vi "Send Batch Messages To Specific Target.vi"(6 "Paras In":variant, 7 "Priority":i32, 8 "error in (no error)":errorcluster, 9 "Mail Strategy In":refnum<class "Mail Strategy.lvclass">, 10 "Messages In":refnum<class "Message.lvclass">[](array[class]), 11 "Map Tree Queue Messenger in":refnum<class "Map Tree Queue Messenger.lvclass">) -> (0 "error out":errorcluster, 3 "Map Tree Queue Messenger out":refnum<class "Map Tree Queue Messenger.lvclass">)   [LabVIEW 2024, in "Map Tree Queue Messenger.lvclass"]
uses:
  Map Tree Queue Messenger.lvclass
  Ancestor Class/Message/Message.lvclass
  Ancestor Class/Messenger/Mail Strategy/Mail Strategy.lvclass
  Mailman/Simple Tree Queue Mailman/Simple Tree Queue Mailman.lvclass
  Ancestor Class/Messenger/Messenger Map Composite/Messenger Map Composite.lvclass/Messenger Map Composite.ctl
  Mailman/Simple Tree Queue Mailman/Simple Tree Queue Mailman.lvclass/Simple Tree Queue Mailman.ctl
  Map Tree Queue Messenger.lvclass/Map Tree Queue Messenger.ctl
  Mailman/Simple Tree Queue Mailman/Public Data/Write Address Recursive Access.vi
  Ancestor Class/Messenger/Messenger Map Composite/Public Data/Read Child Nodes.vi
  Ancestor Class/Messenger/Messenger/Messenger.lvclass
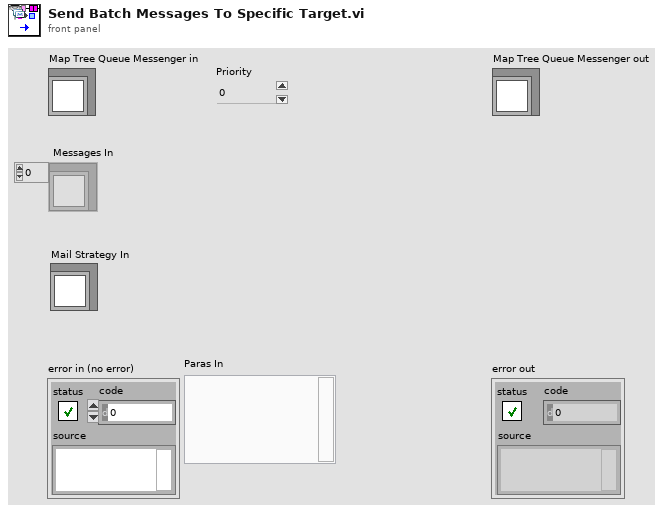
[diagram p1: front panel]
types:
  T1 = typedef "Message Queue.ctl" = refnum<queue>
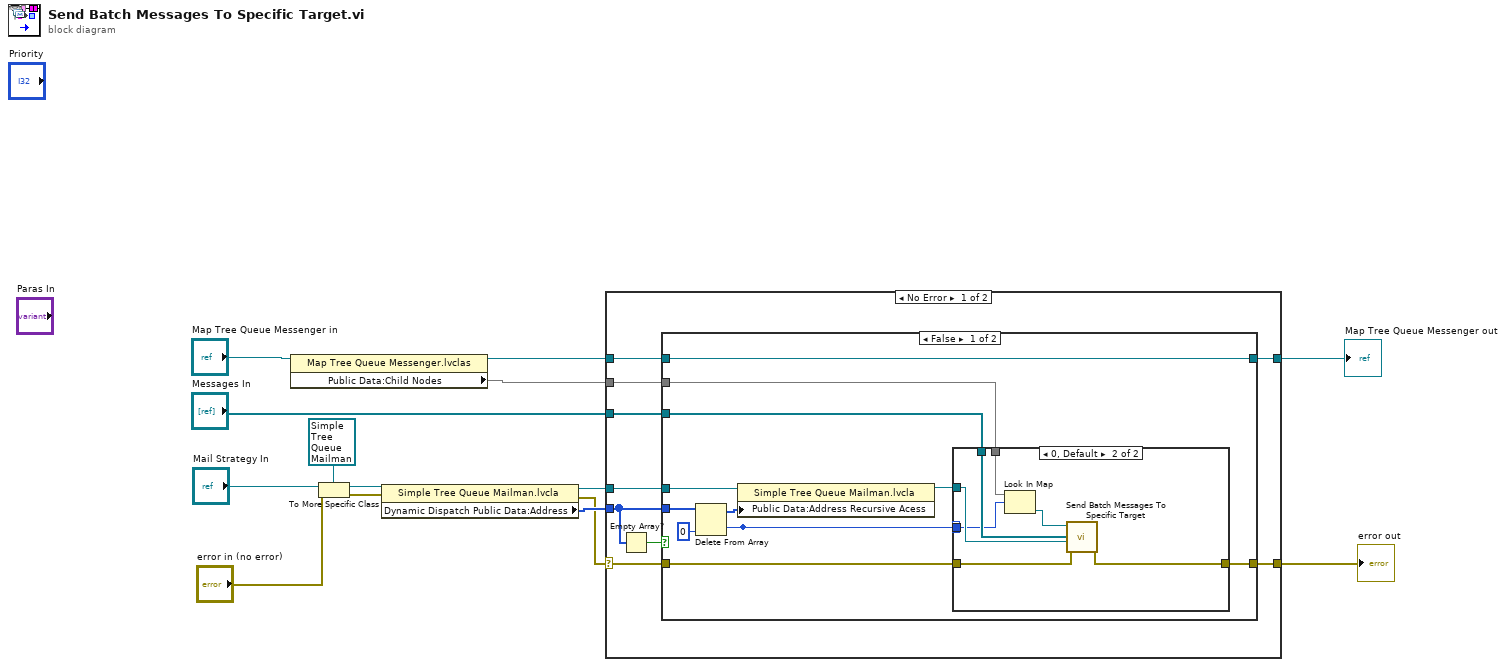
[diagram p0: block diagram]
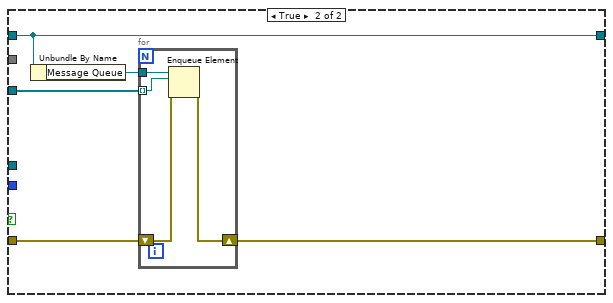
[diagram p3: hidden frame]
diagram:
  n1 = property class="Map Tree Queue Messenger.lvclas"(reference="Map Tree Queue Messenger in") -> (reference out=w9:refnum<class "Map Tree Queue Messenger.lvclass">, "Public Data:Child Nodes"=w8:map{i64, refnum<class "Messenger.lvclass">})  [unwired: 1 in, 1 out]
  n2 = To More Specific Class(target class=refnum<class "Simple Tree Queue Mailman.lvclass"> refnum ("Array Location Mailman.lvclass"), reference="Mail Strategy In", error in="error in (no error)") -> (specific class reference=w12:refnum<class "Simple Tree Queue Mailman.lvclass">, error out=w13:errorcluster)
  n3 = property class="Simple Tree Queue Mailman.lvcla"(reference=w12, error in=w13) -> (reference out=w7:refnum<class "Simple Tree Queue Mailman.lvclass">, error out=w10:errorcluster, "Dynamic Dispatch Public Data:Address"=w11:i32[])
  n4 = case shown="No Error" w10 {
    selector: w10 -> [w18 w52]
    tunnel: w9 -> [w22 w53]
    tunnel: [w20 w53] -> w5
    tunnel: [w17 w52] -> w1
    tunnel: w11 -> [w19 _]
    tunnel: "Messages In" -> [w21 _]
    tunnel: w8 -> [w16 _]
    tunnel: w7 -> [w15 _]
    frame No Error {
      n5 = Empty Array?(array=w19) -> (empty?=w23:bool)
      n6 = case shown="False" w23 {
        tunnel: w22 -> [w34 w47]
        tunnel: w21 -> [w29 w45]
        tunnel: [w34 w47] -> w20
        tunnel: w19 -> [w33 _]
        tunnel: w18 -> [w31 w44]
        tunnel: [w30 w43] -> w17
        tunnel: w16 -> [w28 _]
        tunnel: w15 -> [w27 _]
        frame False {
          n7 = Delete From Array(array=w33, index=0) -> (deleted portion=w24:i32, array with subset deleted=w26:i32[])  [unwired: 1 in]
          n8 = property class="Simple Tree Queue Mailman.lvcla"(reference=w27, "Public Data:Address Recursive Acess"=w26) -> (reference out=w25:refnum<class "Simple Tree Queue Mailman.lvclass">)  [unwired: 1 in, 1 out]
          n9 = case shown="0, Default" w24 {
            tunnel: w24 -> [_ w37]
            tunnel: w31 -> [w35 w42]
            tunnel: [w35 w41] -> w30
            tunnel: w29 -> [_ w40]
            tunnel: w28 -> [_ w38]
            tunnel: w25 -> [_ w39]
            frame -2147483648..-1 {
            }
            frame 0, Default {
              n10 = Look In Map(map=w38, key=w37) -> (value=w36:refnum<class "Messenger.lvclass">)  [unwired: 1 in, 1 out]
              n11 = call-dynamic "Send Batch Messages To Specific Target.vi"("error in (no error)"=w42, "Mail Strategy In"=w39, "Messages In"=w40, "Messenger in"=w36) -> ("error out"=w41:errorcluster)  [unwired: 6 in, 1 out]
            }
          }
        }
        frame True {
          n12 = Unbundle By Name(w47) -> ("Message Queue"=w46:T1)
          n13 = for {
            tunnel: w46 -> [w51]
            tunnel: w45 -> [w50] mode=indexing
            shift-right: [w48] -> w43
            shift-left: w44 -> [w49]
            n14 = Enqueue Element(queue=w51, element=w50, error in (no error)=w49) -> (error out=w48:errorcluster)  [unwired: 1 in, 2 out]
          }
        }
      }
    }
    frame Error {
    }
  }
  "error out" <- w1
  "Map Tree Queue Messenger out" <- w5
